vi "measurementproject.vi"() -> ()   [LabVIEW 2024]
uses:
  <vilib>/Analysis/NI_AALBase.lvlib
  <vilib>/measure/NI_MABase.lvlib
panel:
  in  "Type of wave form":T1(ring)
  in  "Amplitude":dbl(knob) scale=0.0..10.0
  in  "Frequency":dbl(knob) scale=0.0..10.0
  out "Output":waveform(dbl)[](graph)
  out "Input with Noise":waveform(dbl)[](graph)
  in  "stop":bool
  out "Noise Waveform":dbl[](graph)
  in  "Noise Amplitude":dbl=1.0 format="%0.2f"
  in  "Type of Noise":T2(radio)
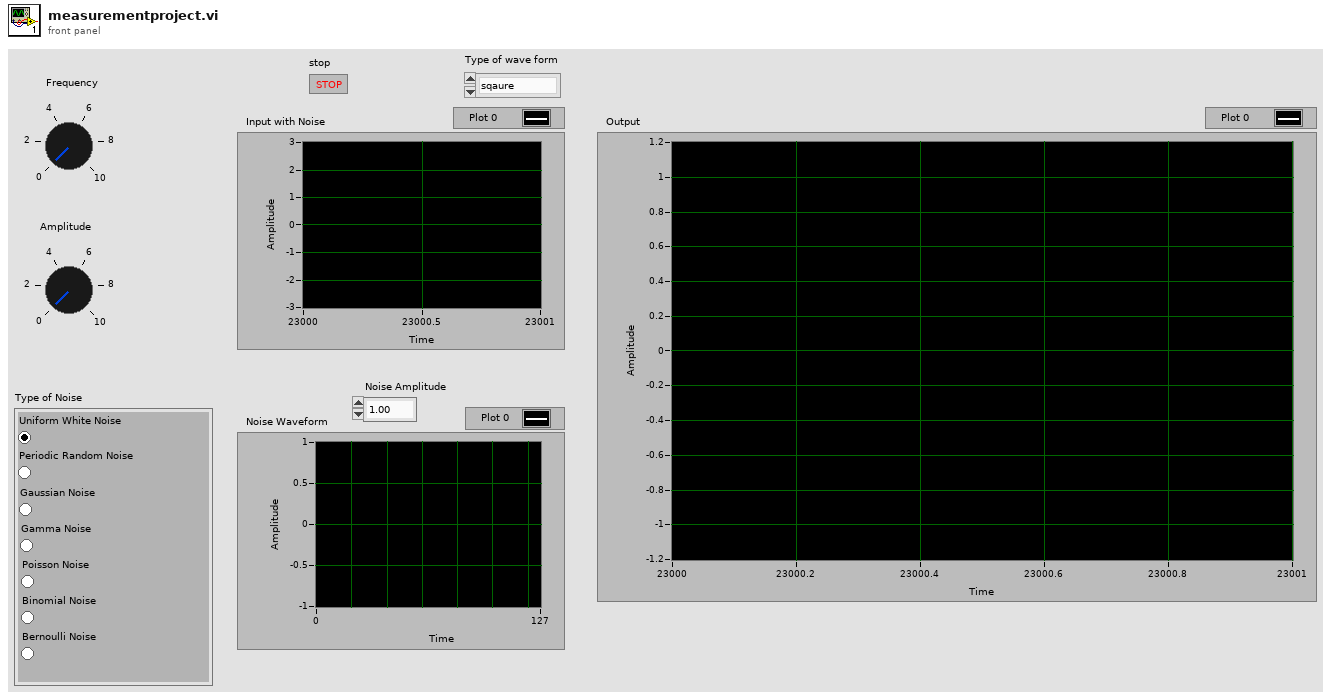
[diagram p1: front panel]
types:
  T1 = enum16{"sqaure", "sine", "triangle", "sawtooth", ""}
  T2 = enum32{"Uniform White Noise", "Periodic Random Noise", "Gaussian Noise", "Gamma Noise", "Poisson Noise", "Binomial Noise", "Bernoulli Noise"}
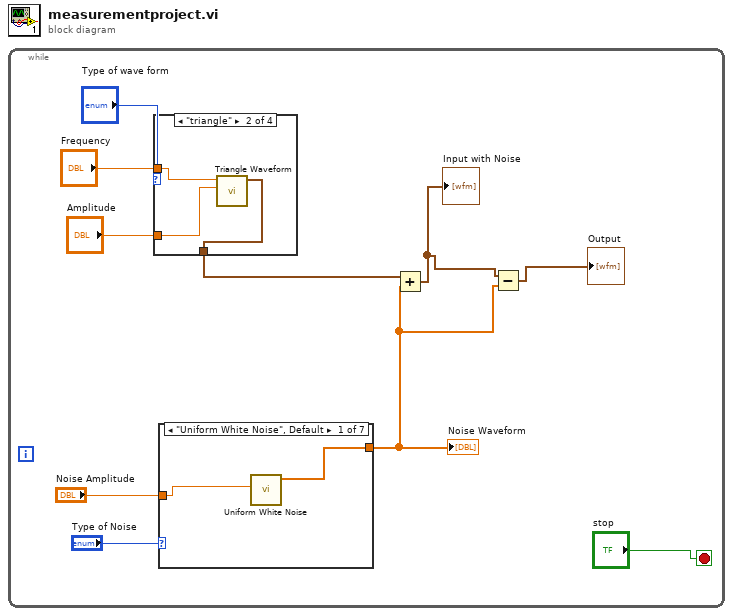
[diagram p0: block diagram]
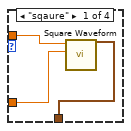
[diagram p2: hidden frame]
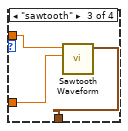
[diagram p3: hidden frame]
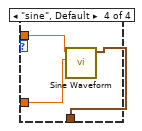
[diagram p4: hidden frame]
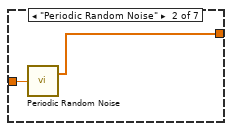
[diagram p5: hidden frame]
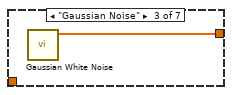
[diagram p6: hidden frame]
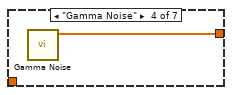
[diagram p7: hidden frame]
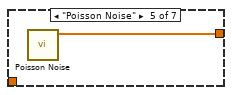
[diagram p8: hidden frame]
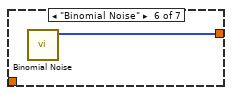
[diagram p9: hidden frame]
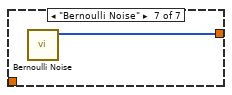
[diagram p10: hidden frame]
diagram:
  n1 = while {
    stop <- "stop" stop-if-true
    n2 = case shown="\"triangle\"" "Type of wave form" {
      tunnel: [w13 w16 w17 w20] -> w7
      tunnel: "Frequency" -> [w12 w15 w19 w22]
      tunnel: "Amplitude" -> [w11 w14 w18 w21]
      frame "sqaure" {
        n3 = call <vilib>:"Square Waveform.vi"("amplitude"=w11, "frequency"=w12) -> ("signal out"=w13:waveform(dbl))  [unwired: 8 in, 1 out]
      }
      frame "triangle" {
        n4 = call <vilib>:"Triangle Waveform.vi"("amplitude"=w14, "frequency"=w15) -> ("signal out"=w16:waveform(dbl))  [unwired: 8 in, 1 out]
      }
      frame "sawtooth" {
        n5 = call <vilib>:"Sawtooth Waveform.vi"("amplitude"=w18, "frequency"=w19) -> ("signal out"=w17:waveform(dbl))  [unwired: 8 in, 1 out]
      }
      frame "sine", Default {
        n6 = call <vilib>:"Sine Waveform.vi"("amplitude"=w21, "frequency"=w22) -> ("signal out"=w20:waveform(dbl))  [unwired: 8 in, 1 out]
      }
    }
    n7 = case shown="\"Uniform White Noise\", Default" "Type of Noise" {
      tunnel: "Noise Amplitude" -> [w24 w26 _ _ _ _ _]
      tunnel: [w23 w25 w27 w28 w29 w30 w31] -> w5
      frame "Uniform White Noise", Default {
        n8 = call <vilib>:"Uniform White Noise.vi"("amplitude"=w24) -> ("uniform white noise"=w23:dbl[])  [unwired: 9 in, 1 out]
      }
      frame "Periodic Random Noise" {
        n9 = call <vilib>:"Periodic Random Noise.vi"("spectral amplitude"=w26) -> ("periodic random noise"=w25:dbl[])  [unwired: 2 in, 1 out]
      }
      frame "Gaussian Noise" {
        n10 = call <vilib>:"Gaussian White Noise.vi"() -> ("Gaussian noise pattern"=w27:dbl[])  [unwired: 10 in, 1 out]
      }
      frame "Gamma Noise" {
        n11 = call <vilib>:"Gamma Noise.vi"() -> ("gamma noise"=w28:dbl[])  [unwired: 10 in, 1 out]
      }
      frame "Poisson Noise" {
        n12 = call <vilib>:"Poisson Noise.vi"() -> ("poisson noise"=w29:dbl[])  [unwired: 10 in, 1 out]
      }
      frame "Binomial Noise" {
        n13 = call <vilib>:"Binomial Noise.vi"() -> ("binomial noise"=w30:u32[])  [unwired: 10 in, 1 out]
      }
      frame "Bernoulli Noise" {
        n14 = call <vilib>:"Bernoulli Noise.vi"() -> ("bernoulli noise"=w31:u8[])  [unwired: 10 in, 1 out]
      }
    }
    "Noise Waveform" <- w5
    n15 = Add(x=w7, y=w5) -> (x+y=w6:waveform(dbl)[])
    "Input with Noise" <- w6
    n16 = Subtract(x=w6, y=w5) -> (x-y=→"Output":waveform(dbl)[])
  }
